vi "Webcam - Initialize Logitech.vi"() -> (0 "error out":errorcluster, 3 "New Image":T1)   [LabVIEW 2011]
uses:
  <vilib>/vision/Image Controls.llb/IMAQ Image.ctl
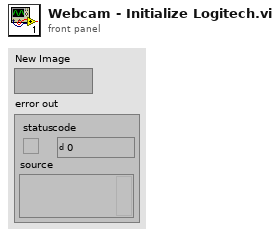
[diagram p1: front panel]
types:
  T1 = typedef "IMAQ Image.ctl" = refnum<image>
  T2 = typedef "Image Type" = u32
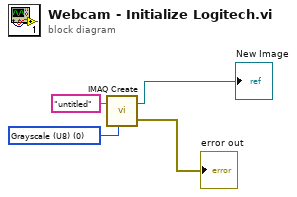
[diagram p0: block diagram]
diagram:
  w3 = T2 0 items=["Grayscale (U8)", "Grayscale (I16)", "Grayscale (SGL)", "Complex (CSG)", "RGB (U32)", "HSL (U32)", "RGB (U64)", "Grayscale (U16)"] ("Image Type")
  n1 = call "IMAQ Create"("Image Name"="untitled", "Image Type"=w3) -> ("New Image"=→"New Image":T1, "error out"=→"error out":errorcluster)  [unwired: 3 in]
